vi "Load.vi"(8 "error in (no error)":errorcluster, 9 "Path":path, 10 "Channel Index":i32, 11 "Mixer in":refnum<class "Mixer.lvclass">) -> (0 "error out":errorcluster, 3 "Mixer out":refnum<class "Mixer.lvclass">)   [LabVIEW 2020, in "G-Audio.lvlib" / "Mixer.lvclass"]
uses:
  Mixer.lvclass
  Mixer.lvclass/Mixer.ctl
  Channel/Load Async.vi
  Channel/Channel.lvclass
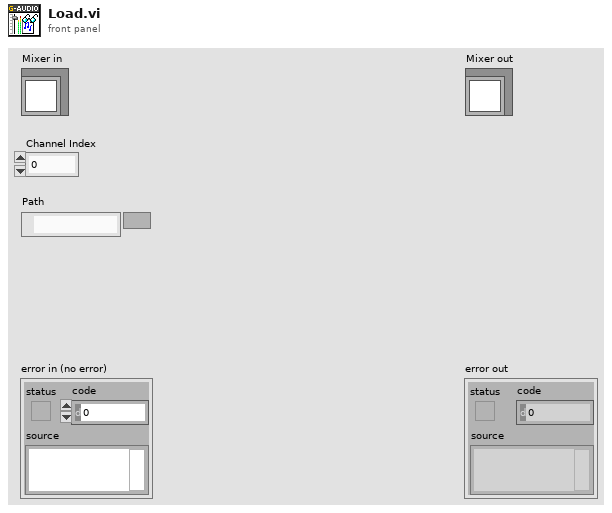
[diagram p1: front panel]
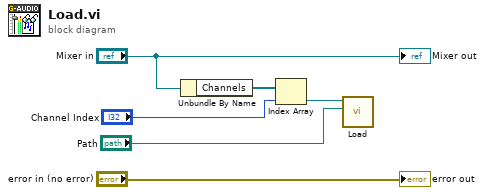
[diagram p0: block diagram]
diagram:
  n1 = Unbundle By Name("Mixer in") -> ("Channels"=w6:refnum<data-value>[])
  n2 = Index Array(array=w6, index="Channel Index") -> (element=w1:refnum<data-value>)
  n3 = call "Load.vi"("Path"="Path", "Channel in"=w1) -> ()  [unwired: 8 in, 2 out]
  "error out" <- "error in (no error)"
  "Mixer out" <- "Mixer in"
